vi "Push_Data_to_Server.vi"(2 "File to Archive":path[](array[path]), 3 "Zip String":string, 4 "Relative Path":path) -> (0 "error out":errorcluster)   [LabVIEW 2011]
uses:
  Anemometry/Anemometry Sub Vis/Globals/Constants_global.vi
  <vilib>/zip/NI_Unzip.lvlib
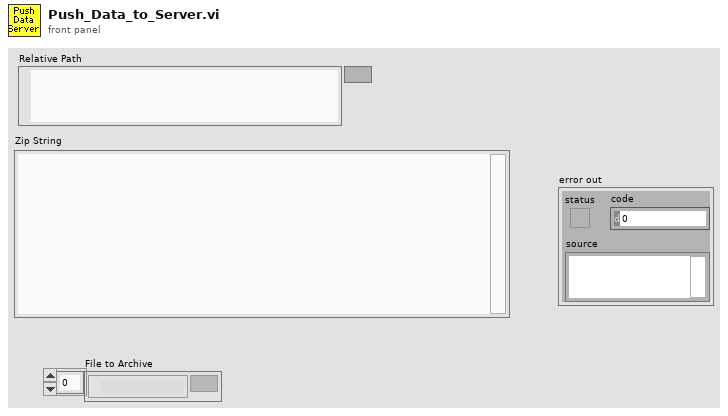
[diagram p1: front panel]
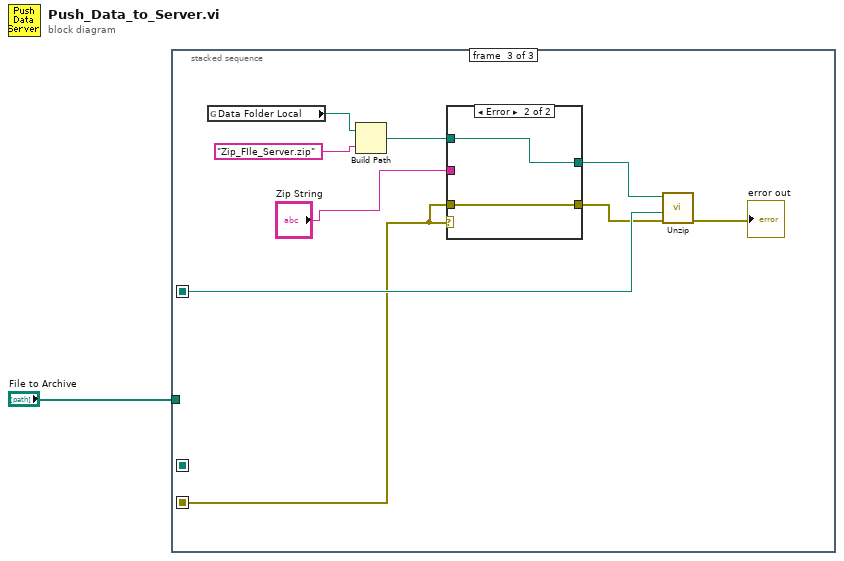
[diagram p0: block diagram]
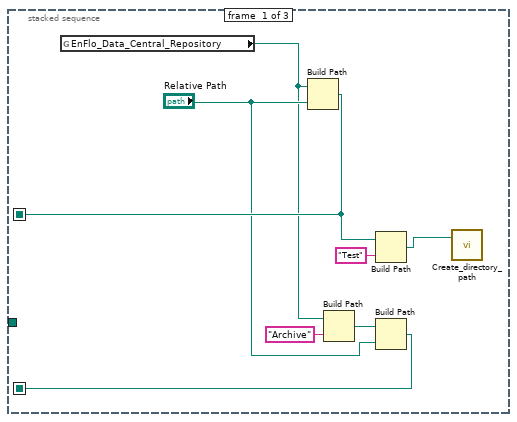
[diagram p2: hidden frame]
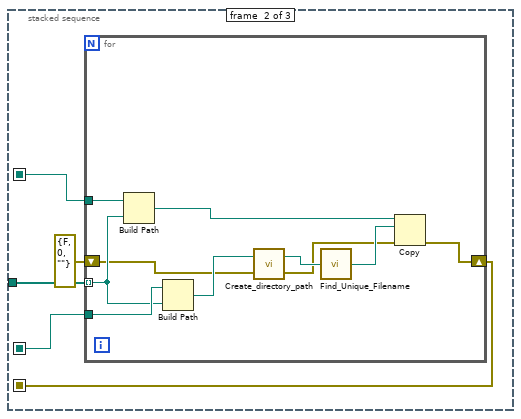
[diagram p3: hidden frame]
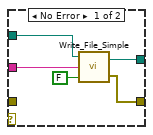
[diagram p4: hidden frame]
diagram:
  n1 = stacked-sequence {
    seq-local: [w7 _ _] -> [_ w12 w30]
    seq-local: [w3 _ _] -> [_ w11 _]
    seq-local: [_ w10 _] -> [_ _ w28]
    tunnel: "File to Archive" -> [_ w14 _]
    frame #0 {
      n2 = global read "Constants_global.vi" "EnFlo_Data_Central_Repository"() -> (w2:path)
      n3 = Build Path(base path=w2, name or relative path="Relative Path") -> (appended path=w7:path)
      n4 = Build Path(base path=w2, name or relative path="Archive") -> (appended path=w5:path)
      n5 = Build Path(base path=w7, name or relative path="Test") -> (appended path=w9:path)
      n6 = Build Path(base path=w5, name or relative path="Relative Path") -> (appended path=w3:path)
      n7 = call "Create_directory_path.vi"("Path name"=w9) -> ()  [unwired: 1 in, 2 out]
    }
    frame #1 {
      n8 = for {
        tunnel: w12 -> [w24]
        tunnel: w14 -> [w21] mode=indexing
        tunnel: w11 -> [w22]
        shift-right: [w20] -> w10
        shift-left: errorcluster {"status"=FALSE, "code"=0, "source"=""} ("error out") -> [w16]
        n9 = Build Path(base path=w24, name or relative path=w21) -> (appended path=w23:path)
        n10 = Build Path(base path=w22, name or relative path=w21) -> (appended path=w18:path)
        n11 = call "Create_directory_path.vi"("error in (no error)"=w16, "Path name"=w18) -> ("error out"=w15:errorcluster, "Path name Out"=w17:path)
        n12 = call "Find_Unique_Filename.vi"("Path In"=w17) -> ("Unique Path Out"=w19:path)  [unwired: 2 in]
        n13 = Copy(8:w15, 10:w19, 11:w23) -> (0:w20:errorcluster)  [unwired: 2 in, 2 out]
      }
    }
    frame #2 {
      n14 = global read "Constants_global.vi" "Data Folder Local"() -> (w32:path)
      n15 = Build Path(base path=w32, name or relative path="Zip_FIle_Server.zip") -> (appended path=w26:path)
      n16 = case shown="Error" w28 {
        tunnel: "Zip String" -> [w38 _]
        tunnel: w28 -> [_ w40]
        tunnel: [w36 w40] -> w27
        tunnel: w26 -> [w35 w39]
        tunnel: [w34 w39] -> w25
        frame No Error {
          n17 = call "Write_File_Simple.vi"("append to file? (new file:F)"=FALSE, "character string"=w38, "file path"=w35) -> ("error out"=w36:errorcluster, "file path Out"=w34:path)
        }
        frame Error {
        }
      }
      n18 = call <vilib>:"Unzip.vi"("error in (no error)"=w27, "Target directory (same as Zip file if empty)"=w30, "Zip file"=w25) -> ("error out"=→"error out":errorcluster)  [unwired: 6 in, 2 out]
    }
  }
